vi "EventBuilder.ProcCases.vi"(0 "i ref in":refnum<vi>, 1 "selector":string, 2 "Data":T1, 3 "call cluster":T2={"Object"="", "Selector"="", "CallType"=enum."synchronous", "Async Object"="", "Async Selector"="", "Data Descriptor"="", "Data"=[], "Error #"=0, "Expire"=0}, 5 "error in (no error)":errorcluster) -> (14 "i ref out":refnum<vi>, 17 "answer cluster":T2={"Object"="", "Selector"="", "CallType"=enum."synchronous", "Async Object"="", "Async Selector"="", "Data Descriptor"="", "Data"=[], "Error #"=0, "Expire"=0}, 19 "error out":errorcluster)   [LabVIEW 2014, in "EventBuilder.lvlib"]
doc: "This method is called by a process from within the default case in the event loop. The methods of a class that are linked to events will be called from THIS method. Add your code here."
uses:
  EventBuilder.lvlib
  CSCore/CSSystem/CoreDefs/CoreDefs.call_type.ctl
  CSCore/BaseProcess/BaseProcess.descriptor string definition.ctl
  CSCore/CSSystem/CoreDefs/CoreDefs.rawDataType.ctl
  CSCore/CSSystem/CoreLib/CoreLib.string 2 byte array.vi
  CSCore/CSSystem/CoreLib/CoreLib.byte array 2 int.vi
  CSCore/CSSystem/CoreLib/CoreLib.byte array 2 string.vi
  CSCore/BaseProcess/BaseProcess.lvlib
  CSCore/CSSystem/CoreLib/CoreLib.lvlib
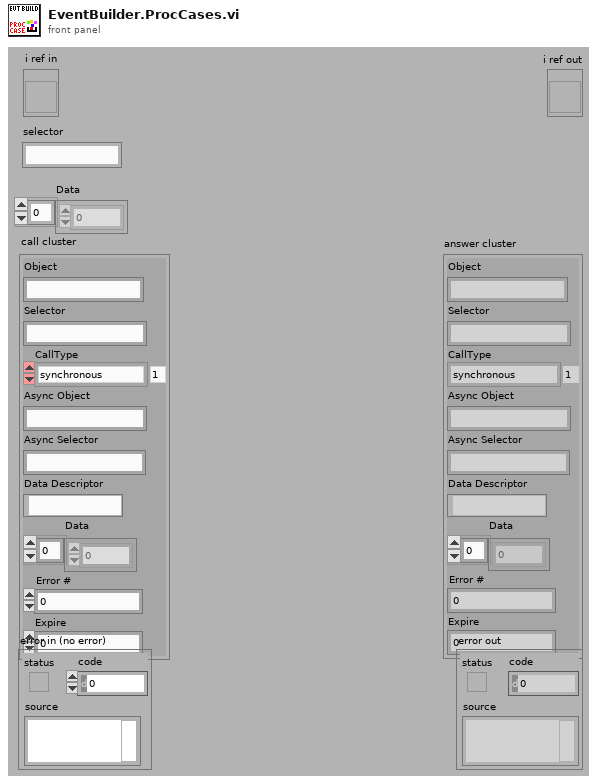
[diagram p1: front panel]
types:
  T1 = typedef "CoreDefs.rawDataType.ctl" = i8[]
  T2 = typedef "CoreDefs.call_type.ctl" = cluster{"Object":string, "Selector":string, "CallType":enum16{"simple", "synchronous", "asynchronous"}, "Async Object":string, "Async Selector":string, "Data Descriptor":T3, "Data":T1, "Error #":i32, "Expire":u32}
  T3 = typedef "BaseProcess.lvlib/BaseProcess.descriptor string definition.ctl" = string
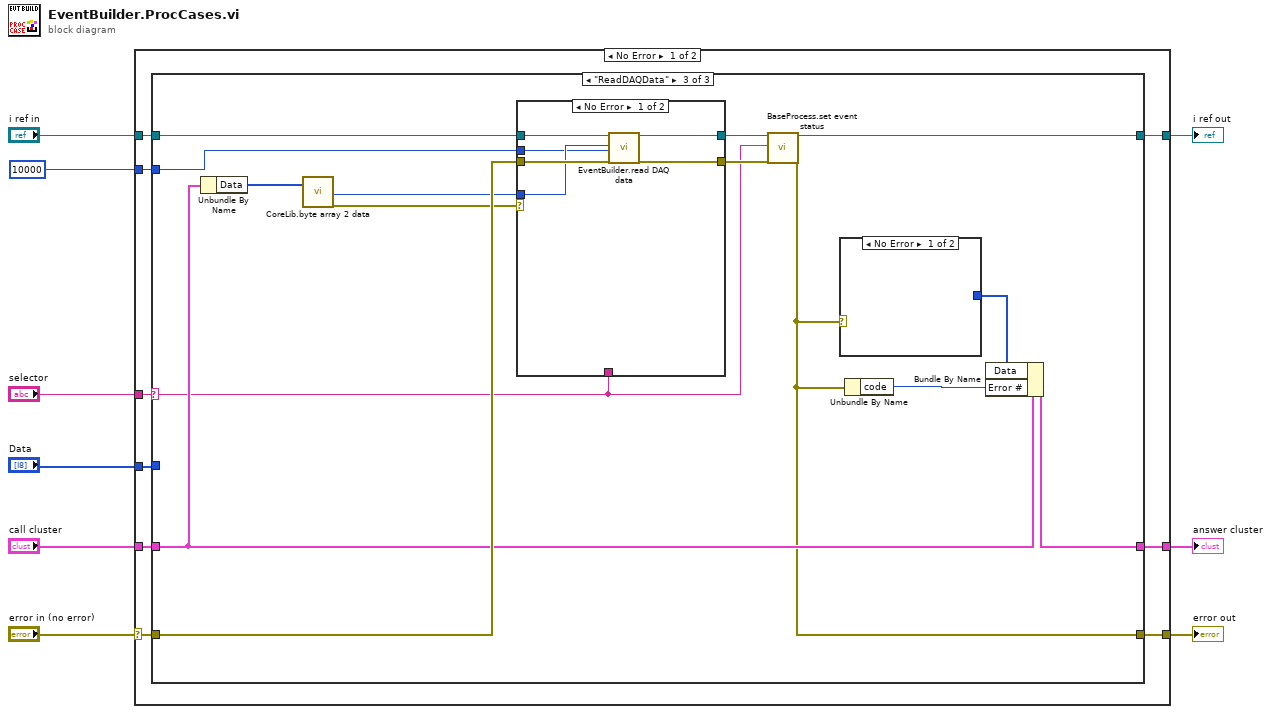
[diagram p0: block diagram]
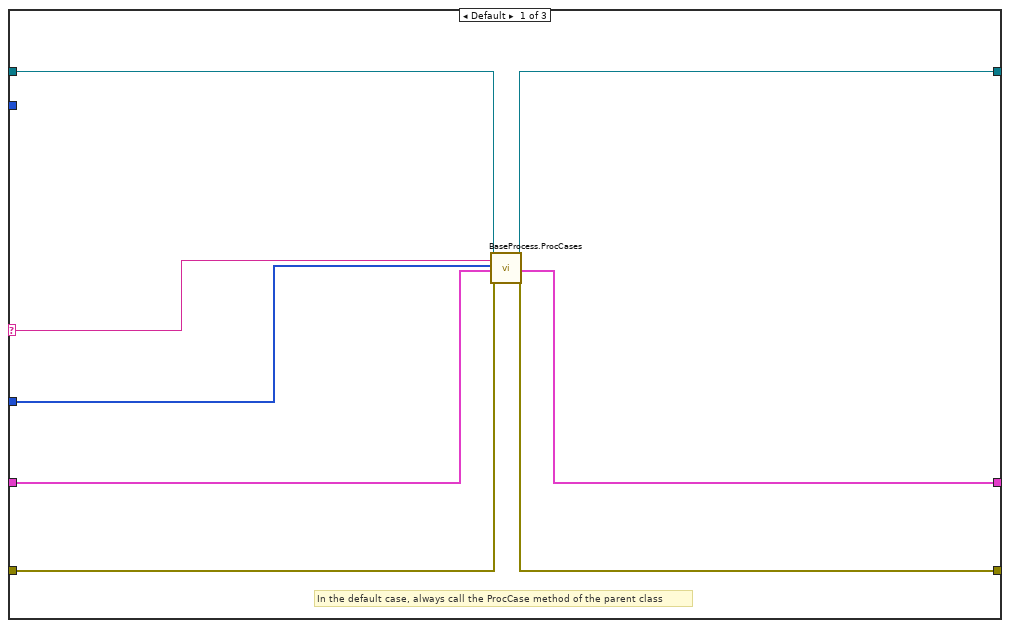
[diagram p2: hidden frame]
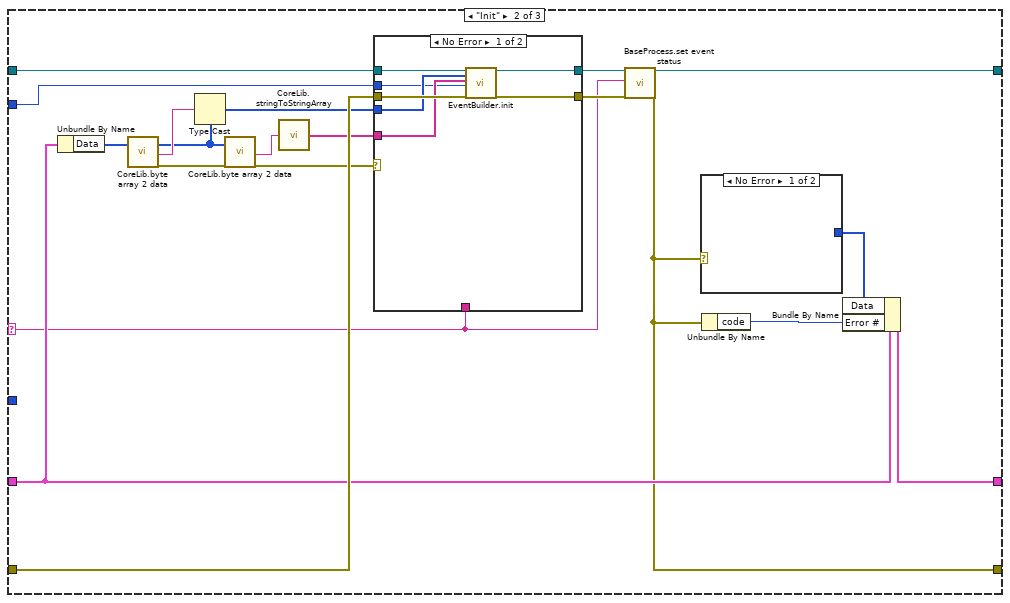
[diagram p3: hidden frame]
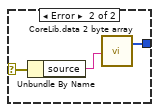
[diagram p4: hidden frame]
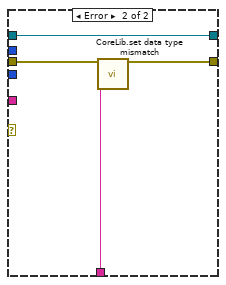
[diagram p5: hidden frame]
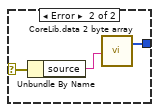
[diagram p6: hidden frame]
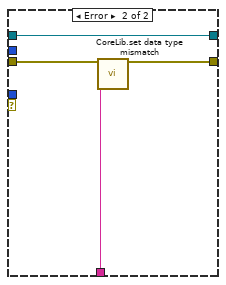
[diagram p7: hidden frame]
diagram:
  n1 = case shown="No Error" "error in (no error)" {
    selector: "error in (no error)" -> [w10 w89]
    tunnel: "selector" -> [w18 _]
    tunnel: [w17 w90] -> w8
    tunnel: "Data" -> [w16 _]
    tunnel: "call cluster" -> [w15 w90]
    tunnel: "i ref in" -> [w14 w91]
    tunnel: [w13 w91] -> w4
    tunnel: [w12 w89] -> w3
    tunnel: 10000 -> [w11 _]
    frame No Error {
      n2 = case shown="\"ReadDAQData\"" w18 {
        selector: w18 -> [w20 w37 w68]
        tunnel: w16 -> [w21 _ _]
        tunnel: w14 -> [w19 w46 w75]
        tunnel: [w26 w36 w67] -> w13
        tunnel: w15 -> [w22 w43 w72]
        tunnel: [w23 w42 w71] -> w17
        tunnel: w10 -> [w25 w45 w74]
        tunnel: [w24 w38 w62] -> w12
        tunnel: w11 -> [_ w35 w66]
        frame Default {
          # "In the default case, always call the ProcCase method of the parent class"
          n3 = call "BaseProcess.ProcCases.vi"("i ref in"=w19, "selector"=w20, "Data"=w21, "call cluster"=w22, "error in (no error)"=w25) -> ("i ref out"=w26:refnum<vi>, "answer cluster"=w23:T2, "error out"=w24:errorcluster)  [unwired: 12 in]
        }
        frame "Init" {
          n4 = Unbundle By Name(w43) -> ("Data"=w34:T1)
          n5 = call-poly "CoreLib.byte array 2 data.vi"("byteArray"=w34) -> ("byteArray out"=w31:T1, "string"=w32:string, "error out"=w33:errorcluster)  [unwired: 16 in]
          n6 = Type Cast(type=w31, x=w32) -> (*(type *) &x=w30:T1)
          n7 = call-poly "CoreLib.byte array 2 data.vi"("byteArray"=w31, "error in (no error)"=w33) -> ("string"=w29:string, "error out"=w28:errorcluster)  [unwired: 15 in, 1 out]
          n8 = call "CoreLib.stringToStringArray.vi"("String"=w29) -> ("Array"=w27:string[])
          n9 = case shown="No Error" w28 {
            tunnel: [w55 w60] -> w40
            tunnel: w46 -> [w56 w60]
            tunnel: w45 -> [w53 w59]
            tunnel: [w54 w58] -> w39
            tunnel: w37 -> [_ w57]
            tunnel: w30 -> [w52 _]
            tunnel: w27 -> [w51 _]
            tunnel: w35 -> [w50 _]
            frame No Error {
              n10 = call "EventBuilder.init.vi"("i ref in"=w56, "header"=w52, "DAQ objects"=w51, "ms timeout (10000)"=w50, "error in (no error)"=w53) -> ("i ref out"=w55:refnum<vi>, "error out"=w54:errorcluster)  [unwired: 12 in, 1 out]
            }
            frame Error {
              n11 = call "CoreLib.set data type mismatch.vi"("error in (no error)"=w59, "error source"=w57) -> ("error out"=w58:errorcluster)  [unwired: 17 in]
            }
          }
          n12 = call "BaseProcess.set event status.vi"("i ref in"=w40, "EventStatus"=w37, "error in (no error)"=w39) -> ("i ref out"=w36:refnum<vi>, "error out"=w38:errorcluster)  [unwired: 14 in, 1 out]
          n13 = case shown="No Error" w38 {
            selector: w38 -> [_ w49]
            tunnel: [_ w47] -> w41
            frame No Error {
            }
            frame Error {
              n14 = Unbundle By Name(w49) -> ("source"=w48:string)
              n15 = call-poly "CoreLib.data 2 byte array.vi"("string"=w48) -> ("byteArray out"=w47:T1)  [unwired: 18 in]
            }
          }
          n16 = Unbundle By Name(w38) -> ("code"=w44:i32)
          n17 = Bundle By Name(cluster=w43, "Data"=w41, "Error #"=w44) -> (w42:T2)
        }
        frame "ReadDAQData" {
          n18 = Unbundle By Name(w72) -> ("Data"=w65:T1)
          n19 = call-poly "CoreLib.byte array 2 data.vi"("byteArray"=w65) -> ("i32"=w63:i32, "error out"=w64:errorcluster)  [unwired: 16 in, 1 out]
          n20 = case shown="No Error" w64 {
            tunnel: [w83 w88] -> w70
            tunnel: w75 -> [w84 w88]
            tunnel: w74 -> [w81 w87]
            tunnel: [w82 w86] -> w69
            tunnel: w68 -> [_ w85]
            tunnel: w63 -> [w80 _]
            tunnel: w66 -> [w79 _]
            frame No Error {
              n21 = call "EventBuilder.read DAQ data.vi"("i ref in"=w84, "eventID"=w80, "ms timeout (10000)"=w79, "error in (no error)"=w81) -> ("i ref out"=w83:refnum<vi>, "error out"=w82:errorcluster)  [unwired: 13 in, 1 out]
            }
            frame Error {
              n22 = call "CoreLib.set data type mismatch.vi"("error in (no error)"=w87, "error source"=w85) -> ("error out"=w86:errorcluster)  [unwired: 17 in]
            }
          }
          n23 = call "BaseProcess.set event status.vi"("i ref in"=w70, "EventStatus"=w68, "error in (no error)"=w69) -> ("i ref out"=w67:refnum<vi>, "error out"=w62:errorcluster)  [unwired: 14 in, 1 out]
          n24 = case shown="No Error" w62 {
            selector: w62 -> [_ w78]
            tunnel: [_ w76] -> w61
            frame No Error {
            }
            frame Error {
              n25 = Unbundle By Name(w78) -> ("source"=w77:string)
              n26 = call-poly "CoreLib.data 2 byte array.vi"("string"=w77) -> ("byteArray out"=w76:T1)  [unwired: 18 in]
            }
          }
          n27 = Unbundle By Name(w62) -> ("code"=w73:i32)
          n28 = Bundle By Name(cluster=w72, "Data"=w61, "Error #"=w73) -> (w71:T2)
        }
      }
    }
    frame Error {
    }
  }
  "answer cluster" <- w8
  "i ref out" <- w4
  "error out" <- w3
